vi "Wr DB ErrorState(boolean).vi"(8 "error in (no error)":errorcluster, 9 "Error PLC boolean":bool[](array[boolean])=[FALSE, FALSE, FALSE, FALSE, FALSE, FALSE, FALSE, FALSE, FALSE, FALSE], 11 "DBlink":string="Driver={ODBC Driver 17 for SQL Server};Server=localhost\\SQLEXPRESS;Database=ZDX201;UID=labview;PWD=Dsa@54137926") -> (0 "error out":errorcluster, 1 "發生error的id":i32[](array[numeric]), 2 "No true":bool=TRUE, 3 "Set true":string)   [LabVIEW 2019]
uses:
  <vilib>/addons/database/Connection.llb/DB Tools Open Connec (String).vi
  <vilib>/addons/database/Connection.llb/Conn Execute.vi
  <vilib>/addons/database/Recordset.llb/Rec Destroy - Connection.vi
  <vilib>/addons/database/NI_Database_API.lvlib
panel:
  out "SetFalse query":string="UPDATE error set state=0 where  id in (1,2,3,4,5,6,7,8,9,10)"
  in  "False SQL query 1":string="UPDATE error set state=0 where  id in ("
  out "SetTrue query":string
  out "No false":bool
  out "Set False":string="1,2,3,4,5,6,7,8,9,10,"
  in  "True SQL query 1":string="UPDATE error set state=1 where  id in ("
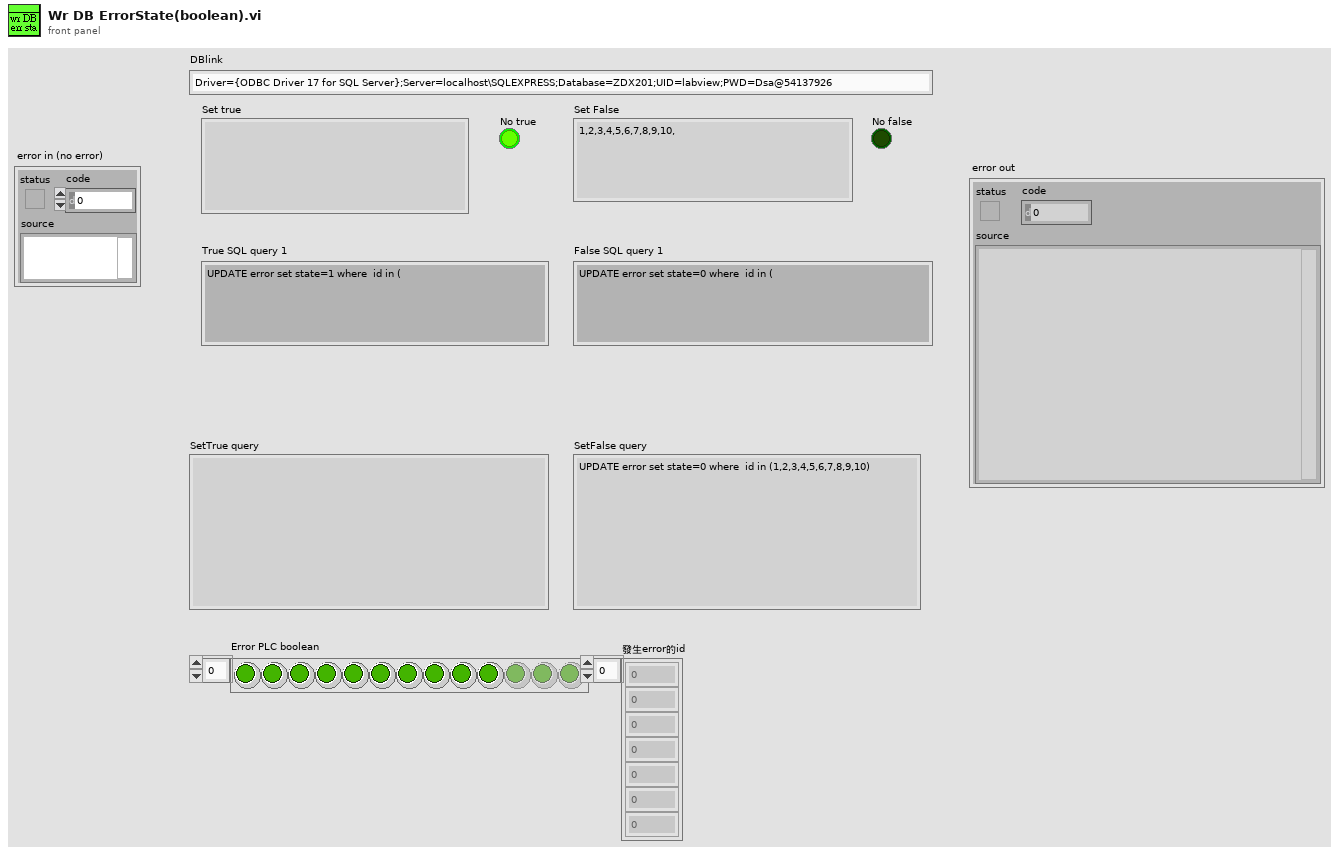
[diagram p1: front panel]
types:
  T1 = typedef "NI_Database_API.lvlib/Conn ObjectReference.ctl" = refnum<k1>
  T2 = typedef "NI_Database_API.lvlib/Rec ObjectReference.ctl" = refnum<k1>
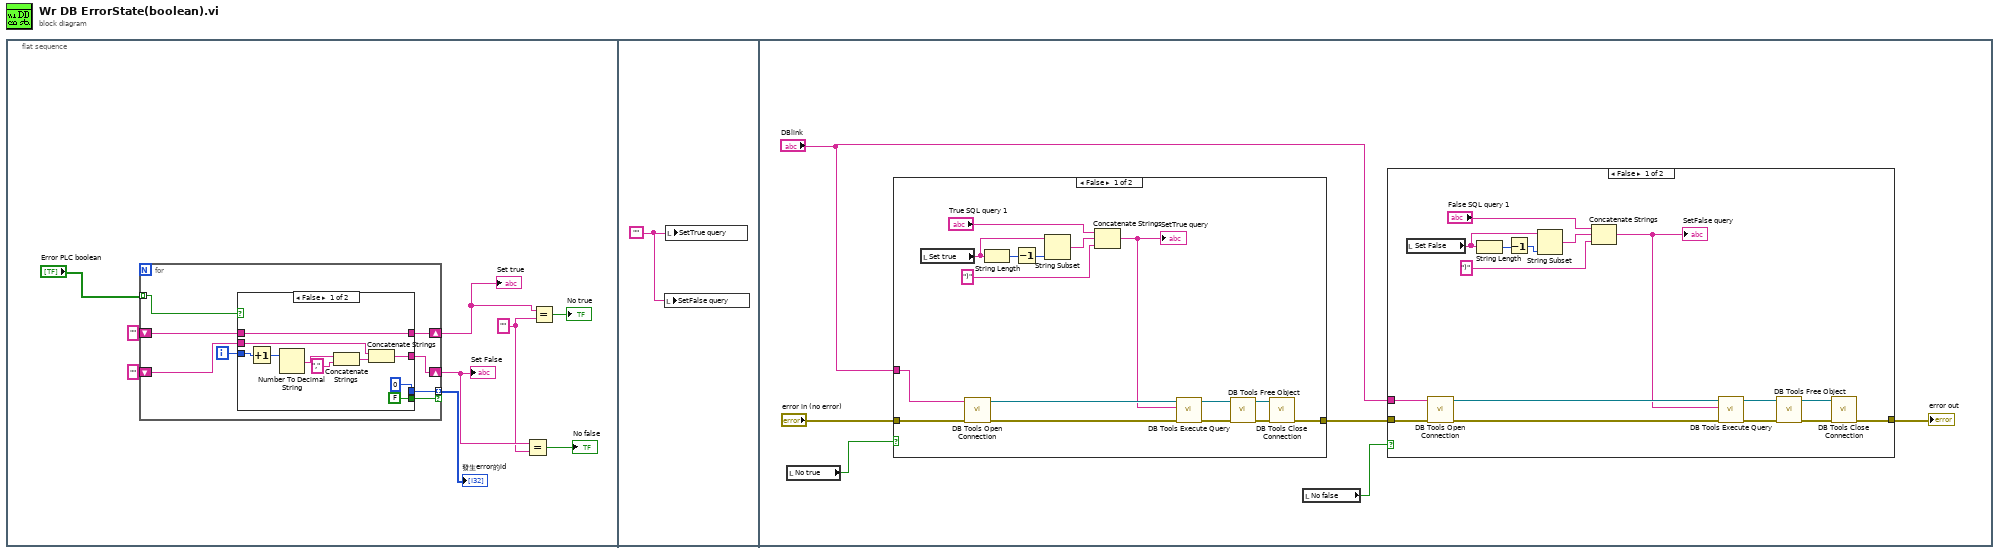
[diagram p0: block diagram]
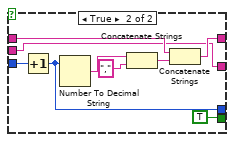
[diagram p2: hidden frame]
diagram:
  n1 = flat-sequence {
    frame #0 {
      w4 = ""
      n2 = for {
        shift-right: [w15] -> w3
        shift-left: "" -> [w16]
        shift-right: [w13] -> w5
        shift-left: "" -> [w14]
        tunnel: "Error PLC boolean" -> [w10] mode=indexing
        tunnel: [w12] -> w2 mode=indexing if=w11
        i -> [w17]
        n3 = case shown="False" w10 {
          tunnel: w17 -> [w25 w36]
          tunnel: w16 -> [w21 w33]
          tunnel: [w21 w32] -> w15
          tunnel: w14 -> [w24 w31]
          tunnel: [w23 w31] -> w13
          tunnel: [0 w29] -> w12
          tunnel: [FALSE TRUE] -> w11
          frame False {
            n4 = Increment(x=w25) -> (x+1=w20:i32)
            n5 = Number To Decimal String(number=w20) -> (decimal integer string=w27:string)  [unwired: 1 in]
            n6 = Concatenate Strings(w27, "," ("string")) -> (w22:string)
            n7 = Concatenate Strings(w24, w22) -> (w23:string)
          }
          frame True {
            n8 = Increment(x=w36) -> (x+1=w29:i32)
            n9 = Number To Decimal String(number=w29) -> (decimal integer string=w35:string)  [unwired: 1 in]
            n10 = Concatenate Strings(w35, "," ("string")) -> (w30:string)
            n11 = Concatenate Strings(w33, w30) -> (w32:string)
          }
        }
      }
      "Set true" <- w3
      "Set False" <- w5
      "發生error的id" <- w2
      n12 = Equal?(x=w5, y=w4) -> (x = y?=→"No false":bool)
      n13 = Equal?(x=w3, y=w4) -> (x = y?=→"No true":bool)
    }
    frame #1 {
      w37 = ""
      n14 = local write "SetFalse query"(w37) -> ()
      n15 = local write "SetTrue query"(w37) -> ()
    }
    frame #2 {
      n16 = local read "No true"() -> (w42:bool)
      n17 = case shown="False" w42 {
        tunnel: "DBlink" -> [w76 _]
        tunnel: [w75 w77] -> w39
        tunnel: "error in (no error)" -> [w72 w77]
        frame False {
          n18 = local read "Set true"() -> (w65:string)
          n19 = call-poly <vilib>:"DB Tools Open Connection.vi"("error in (no error)"=w72, "connection information"=w76) -> ("error out"=w70:errorcluster, "connection reference"=w71:T1)  [unwired: 6 in]
          n20 = String Length(string=w65) -> (length=w67:i32)
          n21 = Decrement(x=w67) -> (x-1=w66:i32)
          n22 = String Subset(string=w65, length (rest)=w66) -> (substring=w64:string)  [unwired: 1 in]
          n23 = Concatenate Strings("True SQL query 1", w64, ")" ("string")) -> (w62:string)
          "SetTrue query" <- w62
          n24 = call-poly <vilib>:"DB Tools Execute Query.vi"("error in (no error)"=w70, "SQL query"=w62, "connection reference"=w71) -> ("error out"=w68:errorcluster, "recordset reference"=w69:T2)  [unwired: 5 in]
          n25 = call-poly <vilib>:"DB Tools Free Object.vi"("error in (no error)"=w68, "recordset reference"=w69) -> ("error out"=w73:errorcluster, "connection reference"=w74:T1)  [unwired: 8 in]
          n26 = call <vilib>:"DB Tools Close Connection.vi"("error in (no error)"=w73, "connection reference"=w74) -> ("error out"=w75:errorcluster)  [unwired: 5 in]
        }
        frame True {
        }
      }
      n27 = local read "No false"() -> (w41:bool)
      n28 = case shown="False" w41 {
        tunnel: "DBlink" -> [w59 _]
        tunnel: [w58 w60] -> w38
        tunnel: w39 -> [w55 w60]
        frame False {
          n29 = local read "Set False"() -> (w46:string)
          n30 = call-poly <vilib>:"DB Tools Open Connection.vi"("error in (no error)"=w55, "connection information"=w59) -> ("error out"=w53:errorcluster, "connection reference"=w54:T1)  [unwired: 6 in]
          n31 = String Length(string=w46) -> (length=w50:i32)
          n32 = Decrement(x=w50) -> (x-1=w49:i32)
          n33 = String Subset(string=w46, length (rest)=w49) -> (substring=w48:string)  [unwired: 1 in]
          n34 = Concatenate Strings("False SQL query 1", w48, ")" ("string")) -> (w45:string)
          "SetFalse query" <- w45
          n35 = call-poly <vilib>:"DB Tools Execute Query.vi"("error in (no error)"=w53, "SQL query"=w45, "connection reference"=w54) -> ("error out"=w51:errorcluster, "recordset reference"=w52:T2)  [unwired: 5 in]
          n36 = call-poly <vilib>:"DB Tools Free Object.vi"("error in (no error)"=w51, "recordset reference"=w52) -> ("error out"=w56:errorcluster, "connection reference"=w57:T1)  [unwired: 8 in]
          n37 = call <vilib>:"DB Tools Close Connection.vi"("error in (no error)"=w56, "connection reference"=w57) -> ("error out"=w58:errorcluster)  [unwired: 5 in]
        }
        frame True {
        }
      }
      "error out" <- w38
    }
  }
